vi "String to Str Hex Array.vi"(8 "error in (no error)":errorcluster, 10 "String":string) -> (0 "error out":errorcluster, 1 "Right":string, 2 "Left":string)   [LabVIEW 2026, in "LED Matrix.lvlib" / "Text.lvclass"]
uses:
  Text.lvclass
  Text.lvclass/Text.ctl
  <vilib>/AdvancedString/1D String Array to Delimited String (string).vi
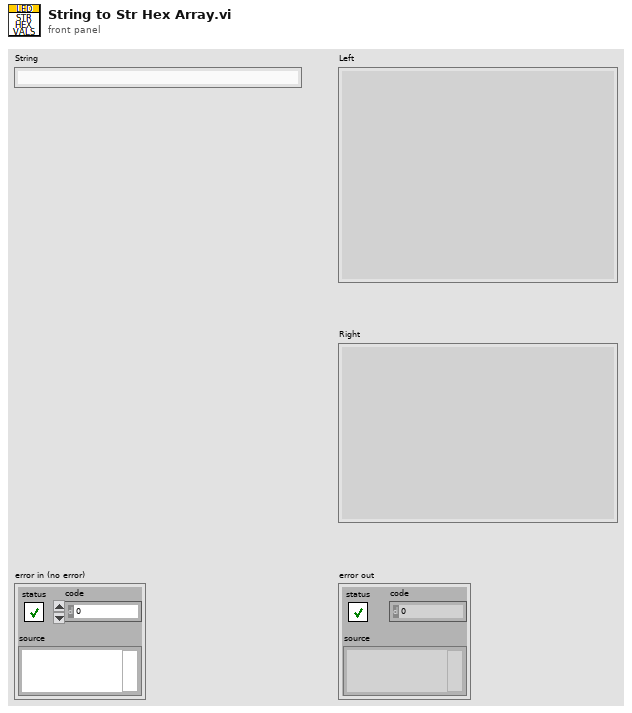
[diagram p1: front panel]
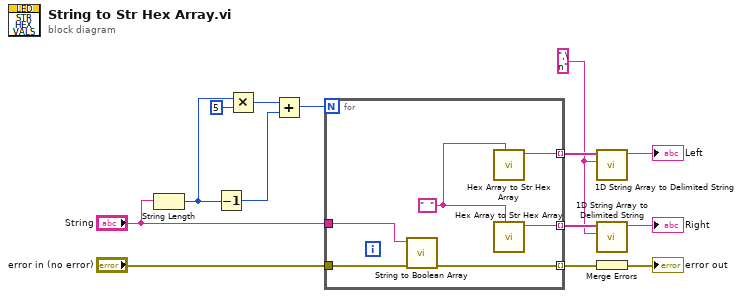
[diagram p0: block diagram]
diagram:
  w1 = ",\n" ("delimiter")
  n1 = String Length(string="String") -> (length=w7:i32)
  n2 = Decrement(x=w7) -> (x-1=w5:i32)
  n3 = Multiply(x=w7, y=5) -> (x*y=w6:i32)
  n4 = Add(x=w6, y=w5) -> (x+y=w4:i32)
  n5 = for {
    N: w4 -> [_]
    tunnel: "error in (no error)" -> [w20]
    tunnel: "String" -> [w15]
    tunnel: [w19] -> w12 mode=indexing
    tunnel: [w18] -> w10 mode=indexing
    tunnel: [w17] -> w9 mode=indexing
    w16 = "  " ("Pre-Line Pad")
    n6 = call "String to Boolean Array.vi"("error in (no error)"=w20, "String"=w15) -> ("error out"=w19:errorcluster)  [unwired: 8 in, 1 out]
    n7 = call "Hex Array to Str Hex Array.vi"("Pre-Line Pad"=w16) -> ("Hex Value String"=w18:string)  [unwired: 10 in]
    n8 = call "Hex Array to Str Hex Array.vi"("Pre-Line Pad"=w16) -> ("Hex Value String"=w17:string)  [unwired: 10 in]
  }
  n9 = call-poly <vilib>:"1D String Array to Delimited String.vi"("delimiter"=w1, "string array"=w10) -> ("delimited string"=→"Left":string)  [unwired: 9 in]
  n10 = call-poly <vilib>:"1D String Array to Delimited String.vi"("delimiter"=w1, "string array"=w9) -> ("delimited string"=→"Right":string)  [unwired: 9 in]
  n11 = Merge Errors(w12) -> (→"error out":errorcluster)
